vi "SetState.vi"(8 "error in":errorcluster, 10 "DLL.state":T1 items=["none", "IR", "LivePL", "PL"], 11 "camera in":refnum<class "camera.lvclass">) -> (0 "error out":errorcluster)   [LabVIEW 2020, in "camera.lvclass"]
uses:
  camera.lvclass
  _controls/DLL.state.ctl
  camera.lvclass/camera.ctl
  lib/O-PL.dll
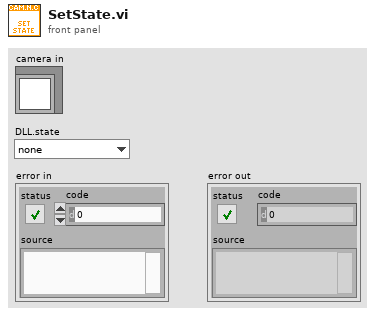
[diagram p1: front panel]
types:
  T1 = typedef "DLL.state.ctl" = u16
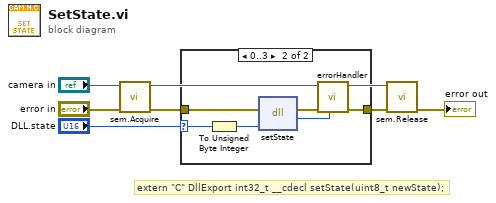
[diagram p0: block diagram]
diagram:
  # "extern \"C\" DllExport int32_t __cdecl setState(uint8_t newState);"
  n1 = call "sem.Acquire.vi"("error in"="error in", "camera.nit in"="camera in") -> ("error out"=w6:errorcluster)  [unwired: 9 in]
  n2 = case shown="0..3" "DLL.state" {
    selector: "DLL.state" -> [_ w11]
    tunnel: w6 -> [w7 w13]
    tunnel: [w7 w8] -> w5
    frame Default {
    }
    frame 0..3 {
      n3 = To Unsigned Byte Integer(number=w11) -> (unsigned 8bit integer=w12:u8)
      n4 = dll-call lib="C:/Users/pittsburger.SOLARIS/Desktop/v0.8/lib/O-PL.dll" fn="setState"(error in=w13, "newState"=w12) -> (error out=w10:errorcluster, "return"=w9:i32)  [unwired: 3 in, 1 out]
      n5 = call "errorHandler.vi"("code"=w9, "error in"=w10) -> ("error out"=w8:errorcluster)  [unwired: 9 in]
    }
  }
  n6 = call "sem.Release.vi"("error in"=w5, "camera.nit in"="camera in") -> ("error out"=→"error out":errorcluster)  [unwired: 9 in]
